vi "Init.vi"(8 "error in (no error)":errorcluster, 11 "Keithley230X in":refnum<class "Keithley230X.lvclass">) -> (0 "error out":errorcluster, 3 "Keithley230X out":refnum<class "Keithley230X.lvclass">)   [LabVIEW 2020, in "LAF2024Q2.lvlib" / "Keithley230X.lvclass"]
uses:
  Keithley230X.lvclass
  C:/dev/lv20CE/LAF2024Q2/LAF2024Q2/PowerSupplyVisa/PowerSupplyVisa.lvclass
  C:/dev/lv20CE/LAF2024Q2/LAF2024Q2/PowerSupply/PowerSupply.lvclass
  PowerSupplyVisa/PowerSupplyVisa.lvclass
  PowerSupply/PowerSupply.lvclass
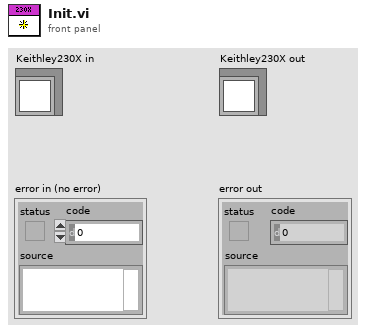
[diagram p1: front panel]
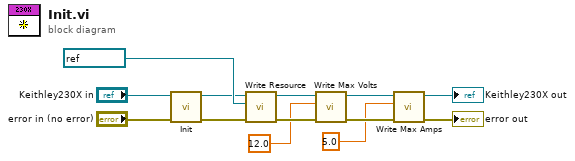
[diagram p0: block diagram]
diagram:
  n1 = call-parent "Init.vi"("error in (no error)"="error in (no error)", "PowerSupply in"="Keithley230X in") -> ("error out"=w3:errorcluster, "PowerSupply out"=w1:refnum<class "Keithley230X.lvclass">)  [unwired: 8 in]
  n2 = call "Write Resource.vi"("error in (no error)"=w3, "Resource"=refnum<visa-resource-name> "COM2", "PowerSupplyVisa in"=w1) -> ("error out"=w12:errorcluster, "PowerSupplyVisa out"=w9:refnum<class "Keithley230X.lvclass">)  [unwired: 7 in]
  n3 = call "Write Max Volts.vi"("error in (no error)"=w12, "Max Voltage"=12.0, "PowerSupply in"=w9) -> ("error out"=w10:errorcluster, "PowerSupply out"=w6:refnum<class "Keithley230X.lvclass">)  [unwired: 7 in]
  n4 = call "Write Max Amps.vi"("error in (no error)"=w10, "Max Current"=5.0, "PowerSupply in"=w6) -> ("error out"=→"error out":errorcluster, "PowerSupply out"=→"Keithley230X out":refnum<class "Keithley230X.lvclass">)  [unwired: 7 in]
